vi "GlobalGetAvantesSpectrometerOnOff.vi"() -> ()   [LabVIEW 2011]
panel:
  out "GetAvantes":bool
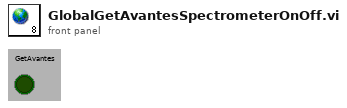
[diagram p1: front panel]
diagram:
